vi "Camera State.vi"(7 "Get/Set":enum16{"Get", "Set"}(ring), 8 "error in (no error)":errorcluster, 9 "Camera Name":string, 10 "New State":T1, 11 "FlexWorktable in":refnum<class "FlexWorktable.lvclass">) -> (0 "error out":errorcluster, 2 "State":T1, 3 "FlexWorktable out":refnum<class "FlexWorktable.lvclass">)   [LabVIEW 2017, in "FlexWorktable.lvclass"]
uses:
  FlexWorktable.lvclass
  Camera State.ctl
  Utils/Geometry Utils/Camera Rotation.ctl
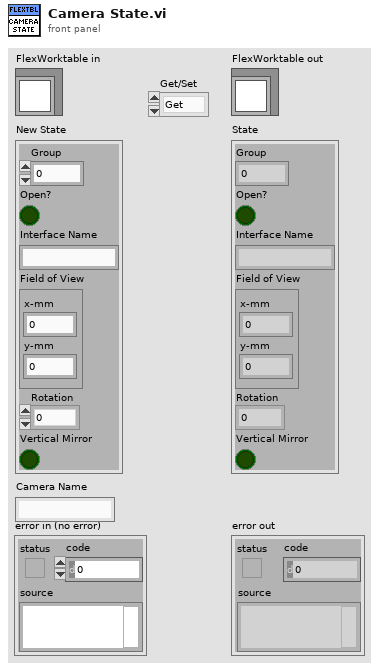
[diagram p1: front panel]
types:
  T1 = typedef "FlexWorktable.lvclass/Camera State.ctl" = cluster{"Group":i32, "Open?":bool, "Interface Name":string, "Field of View":cluster{"x-mm":dbl, "y-mm":dbl}, "Rotation":T2, "Vertical Mirror":bool}
  T2 = typedef "Camera Rotation.ctl" = enum16{"0", "90", "180", "270"}
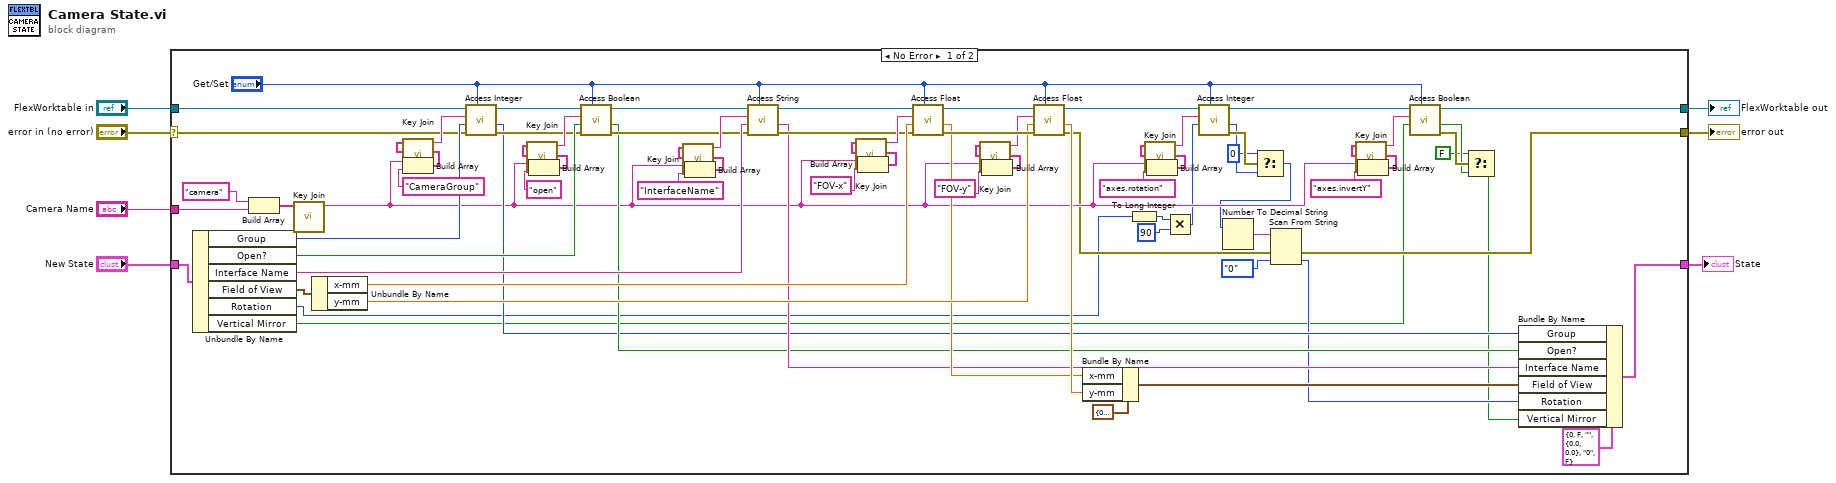
[diagram p0: block diagram]
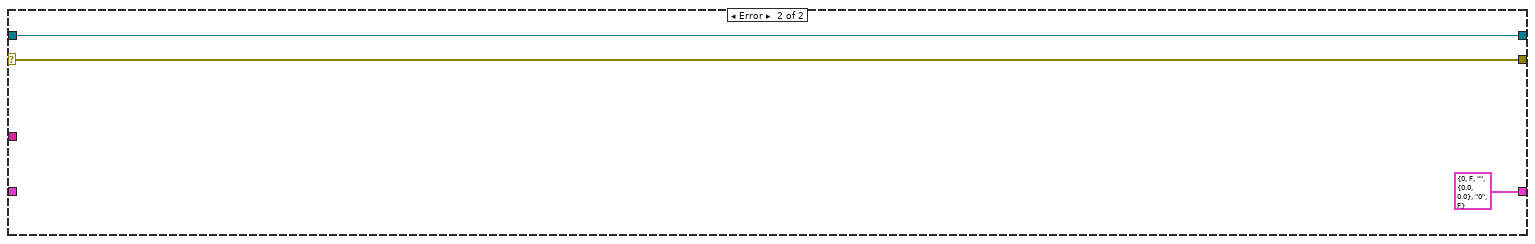
[diagram p2: hidden frame]
diagram:
  n1 = case shown="No Error" "error in (no error)" {
    selector: "error in (no error)" -> [w37 w83]
    tunnel: [w17 w83] -> w6
    tunnel: [w22 w82] -> w4
    tunnel: "FlexWorktable in" -> [w78 w82]
    tunnel: "New State" -> [w80 _]
    tunnel: "Camera Name" -> [w74 _]
    tunnel: [w38 T1 {"Group"=0, "Open?"=FALSE, "Interface Name"="", "Field of View"={"x-mm"=0.0, "y-mm"=0.0}, "Rotation"=enum."0", "Vertical Mirror"=FALSE} ("New State")] -> w1
    frame No Error {
      n2 = Unbundle By Name(w80) -> ("Group"=w77:i32, "Open?"=w66:bool, "Interface Name"=w61:string, "Field of View"=w79:cluster{"x-mm":dbl, "y-mm":dbl}, "Rotation"=w11:T2, "Vertical Mirror"=w9:bool)
      n3 = Build Array("camera", w74) -> (w76:string[])
      n4 = call "Key Join.vi"("Key Elements"=w76) -> ("Key"=w21:string)  [unwired: 10 in]
      n5 = Unbundle By Name(w79) -> ("x-mm"=w56:dbl, "y-mm"=w47:dbl)
      n6 = Build Array(w21, "CameraGroup") -> (w72:string[])
      n7 = call "Key Join.vi"("Key Elements"=w72) -> ("Key"=w71:string)  [unwired: 10 in]
      n8 = call-dynamic "Access Integer.vi"("Get/Set"="Get/Set", "error in (no error)"=w37, "Value in"=w77, "Key"=w71, "FlexWorktable in"=w78) -> ("error out"=w55:errorcluster, "Value out"=w39:i32, "FlexWorktable out"=w68:refnum<class "FlexWorktable.lvclass">)  [unwired: 4 in]
      n9 = Build Array(w21, "open") -> (w69:string[])
      n10 = call "Key Join.vi"("Key Elements"=w69) -> ("Key"=w67:string)  [unwired: 10 in]
      n11 = call-dynamic "Access Boolean.vi"("Get/Set"="Get/Set", "error in (no error)"=w55, "Value in"=w66, "Key"=w67, "FlexWorktable in"=w68) -> ("error out"=w54:errorcluster, "Value out"=w40:bool, "FlexWorktable out"=w63:refnum<class "FlexWorktable.lvclass">)  [unwired: 4 in]
      n12 = Build Array(w21, "InterfaceName") -> (w64:string[])
      n13 = call "Key Join.vi"("Key Elements"=w64) -> ("Key"=w62:string)  [unwired: 10 in]
      n14 = call-dynamic "Access String.vi"("Get/Set"="Get/Set", "error in (no error)"=w54, "Value in"=w61, "Key"=w62, "FlexWorktable in"=w63) -> ("error out"=w53:errorcluster, "Value out"=w41:string, "FlexWorktable out"=w57:refnum<class "FlexWorktable.lvclass">)  [unwired: 4 in]
      n15 = Build Array(w21, "FOV-x") -> (w59:string[])
      n16 = call "Key Join.vi"("Key Elements"=w59) -> ("Key"=w58:string)  [unwired: 10 in]
      n17 = call-dynamic "Access Float.vi"("Get/Set"="Get/Set", "error in (no error)"=w53, "Value in"=w56, "Key"=w58, "FlexWorktable in"=w57) -> ("error out"=w51:errorcluster, "Value out"=w42:dbl, "FlexWorktable out"=w52:refnum<class "FlexWorktable.lvclass">)  [unwired: 4 in]
      n18 = Build Array(w21, "FOV-y") -> (w49:string[])
      n19 = call "Key Join.vi"("Key Elements"=w49) -> ("Key"=w48:string)  [unwired: 10 in]
      n20 = call-dynamic "Access Float.vi"("Get/Set"="Get/Set", "error in (no error)"=w51, "Value in"=w47, "Key"=w48, "FlexWorktable in"=w52) -> ("error out"=w18:errorcluster, "Value out"=w43:dbl, "FlexWorktable out"=w33:refnum<class "FlexWorktable.lvclass">)  [unwired: 4 in]
      n21 = Bundle By Name(cluster=cluster{"x-mm":dbl, "y-mm":dbl} {"x-mm"=0.0, "y-mm"=0.0} ("Field of View"), "x-mm"=w42, "y-mm"=w43) -> (w44:cluster{"x-mm":dbl, "y-mm":dbl})
      n22 = To Long Integer(number=w11) -> (32bit integer=w13:i32)
      n23 = Build Array(w21, "axes.rotation") -> (w35:string[])
      n24 = call "Key Join.vi"("Key Elements"=w35) -> ("Key"=w34:string)  [unwired: 10 in]
      n25 = Multiply(x=w13, y=90) -> (x*y=w10:i32)
      n26 = call-dynamic "Access Integer.vi"("Get/Set"="Get/Set", "Value in"=w10, "Key"=w34, "FlexWorktable in"=w33) -> ("error out"=w32:errorcluster, "Value out"=w31:i32, "FlexWorktable out"=w25:refnum<class "FlexWorktable.lvclass">)  [unwired: 5 in]
      n27 = Select(t=0, s=w32, f=w31) -> (s? t:f=w8:i32)
      n28 = Number To Decimal String(number=w8) -> (decimal integer string=w20:string)  [unwired: 1 in]
      n29 = Scan From String(input string=w20, error in=w18, default 1=Camera_Rotation."0" ("Rotation")) -> (error out=w17:errorcluster, output 1=w16:T2)  [unwired: 2 in, 2 out]
      n30 = Build Array(w21, "axes.invertY") -> (w28:string[])
      n31 = call "Key Join.vi"("Key Elements"=w28) -> ("Key"=w27:string)  [unwired: 10 in]
      n32 = call-dynamic "Access Boolean.vi"("Get/Set"="Get/Set", "Value in"=w9, "Key"=w27, "FlexWorktable in"=w25) -> ("error out"=w26:errorcluster, "Value out"=w24:bool, "FlexWorktable out"=w22:refnum<class "FlexWorktable.lvclass">)  [unwired: 5 in]
      n33 = Select(t=FALSE, s=w26, f=w24) -> (s? t:f=w15:bool)
      n34 = Bundle By Name(cluster=T1 {"Group"=0, "Open?"=FALSE, "Interface Name"="", "Field of View"={"x-mm"=0.0, "y-mm"=0.0}, "Rotation"=enum."0", "Vertical Mirror"=FALSE} ("State 2"), "Group"=w39, "Open?"=w40, "Interface Name"=w41, "Field of View"=w44, "Rotation"=w16, "Vertical Mirror"=w15) -> (w38:T1)
    }
    frame Error {
    }
  }
  "error out" <- w6
  "FlexWorktable out" <- w4
  "State" <- w1
